vi "Init - Core.vi"(8 "error in (no error)":errorcluster, 11 "Error Filter in":refnum<class "Error Filter.lvclass">) -> (0 "error out":errorcluster, 3 "Error Filter out":refnum<class "Error Filter.lvclass">)   [LabVIEW 2026, in "TALOS.lvlib" / "Classes.lvlib" / "Error Filter.lvclass"]
uses:
  Error Filter.lvclass
  Error Filter Properties.ctl
  Ancestor/Ancestor/Ancestor.lvclass/Ancestor.ctl
  Error Filter.lvclass/Error Filter.ctl
  Support VIs/Generate Error.vi
  FGV/Error Memory/Get Error Description.vi
  Support VIs/Get PC name.vi
  Ancestor/Ancestor/Read ID.vi
  Support VIs/Get Class Name.vi
  <vilib>/Utility/error.llb/Clear Errors.vi
  FGV/Error Memory/Error Memory Core.vi
  <vilib>/AdvancedString/Delimited String to 1D String Array.vi
  <vilib>/AdvancedString/Delimited String to 1D String Array (string).vi
  Support VIs/Circus Root Path.vi
  FGV/Error Memory/Error Crt Lvl checker.vi
  FGV/Error Memory/Error Memory Core.vi/40c8088d-b597-4017-91af-faa98e00292e.vi
  FGV/Error Memory/Error Memory Core.vi/d4a3ab98-063c-4e44-b43d-fbdcfe6c2be2.vi
  Support VIs/Global Memory.vi
  <vilib>/Utility/LVClass/Get LV Class Name.vi
  Support VIs/Is in Packed Library.vi
  Support VIs/TALOS Root path.vi
  Support VIs/Read CSV worksheet.vi
  Support VIs/Global Constants.vi
  <vilib>/Utility/error.llb/General Error Handler.vi
  <vilib>/Utility/config.llb/Open Config Data.vi
  <vilib>/Utility/config.llb/Get Section Names.vi
  <vilib>/Utility/config.llb/Get Key Names.vi
  <vilib>/Utility/config.llb/Read Key.vi
  <vilib>/Utility/config.llb/Read Key (String).vi
  <vilib>/Utility/config.llb/Close Config Data.vi
  Ancestor/Ancestor/Ancestor.lvclass
  <vilib>/Comparison/Equal/Equal Functor/Equal Functor.lvclass
  TALOS.lvlib
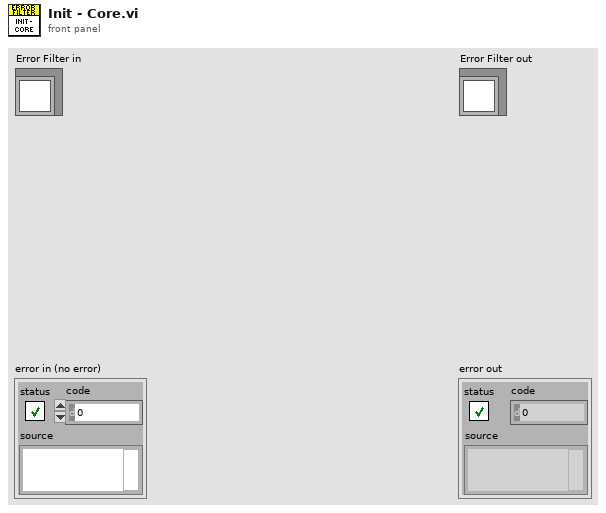
[diagram p1: front panel]
types:
  T1 = typedef "TALOS.lvlib/Classes.lvlib/Error Filter.lvclass/Error Filter Properties.ctl" = cluster{"Repetitions":u32, "Until":timestamp}
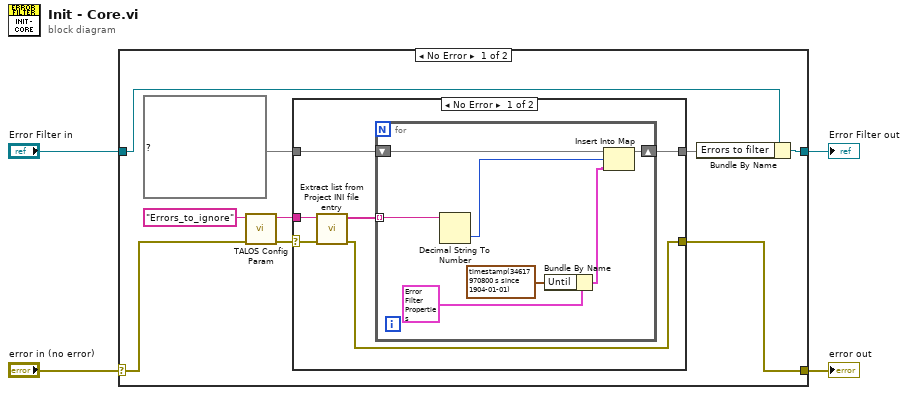
[diagram p0: block diagram]
diagram:
  n1 = case shown="No Error" "error in (no error)" {
    selector: "error in (no error)" -> [w12 w30]
    tunnel: [w10 w30] -> w3
    tunnel: [w6 w29] -> w1
    tunnel: "Error Filter in" -> [w7 w29]
    frame No Error {
      n2 = call "TALOS Config Param.vi"("error in (no error)"=w12, "Parameter Name"="Errors_to_ignore") -> ("error out"=w11:errorcluster, "Output"=w9:string)  [unwired: 8 in]
      n3 = case shown="No Error" w11 {
        selector: w11 -> [w17 w28]
        tunnel: [w16 w28] -> w10
        tunnel: w9 -> [w15 _]
        tunnel: map{i32, T1} {} ("Errors to filter") -> [w19 w27]
        tunnel: [w18 w27] -> w5
        frame No Error {
          n4 = call "Extract list from Project INI file entry.vi"("error in (no error)"=w17, "Entry from INI file"=w15) -> ("error out"=w16:errorcluster, "Array"=w14:string[])  [unwired: 8 in]
          n5 = for {
            shift-right: [w25] -> w18
            shift-left: w19 -> [w26]
            tunnel: w14 -> [w20] mode=indexing
            n6 = Decimal String To Number(string=w20) -> (number=w24:i32)  [unwired: 2 in, 1 out]
            n7 = Bundle By Name(cluster=T1 {"Repetitions"=1, "Until"=timestamp(0 s since 1904-01-01)} ("value"), "Until"=timestamp(34617970800 s since 1904-01-01)) -> (w22:T1)
            n8 = Insert Into Map(map in=w26, key=w24, value=w22) -> (map out=w25:map{i32, T1})  [unwired: 2 out]
          }
        }
        frame Error {
        }
      }
      n9 = Bundle By Name(cluster=w7, "Errors to filter"=w5) -> (w6:refnum<class "Error Filter.lvclass">)
    }
    frame Error {
    }
  }
  "error out" <- w3
  "Error Filter out" <- w1
